vi "Estrazione.vi"(0 "Percorso file invenduti (se vuoto finestra di dialogo)":path) -> (1 "Ci sono numeri estratti invenduti!!!":bool, 2 "Numeri estratti":i32[](array[numeric]))   [LabVIEW 2012]
uses:
  <vilib>/Utility/file.llb/Write To Spreadsheet File (I64).vi
  <vilib>/Utility/file.llb/Read From Spreadsheet File (I64).vi
panel:
  in  "Numero massimo\nvenduto":i32=5000
  in  "Quanti numeri estrarre":i32=25
  out "Numeri invenduti":i64[](array[numeric])
  out "Numeri estratti senza\ncontrollo":i32[](array[numeric]) format="%#.0f"
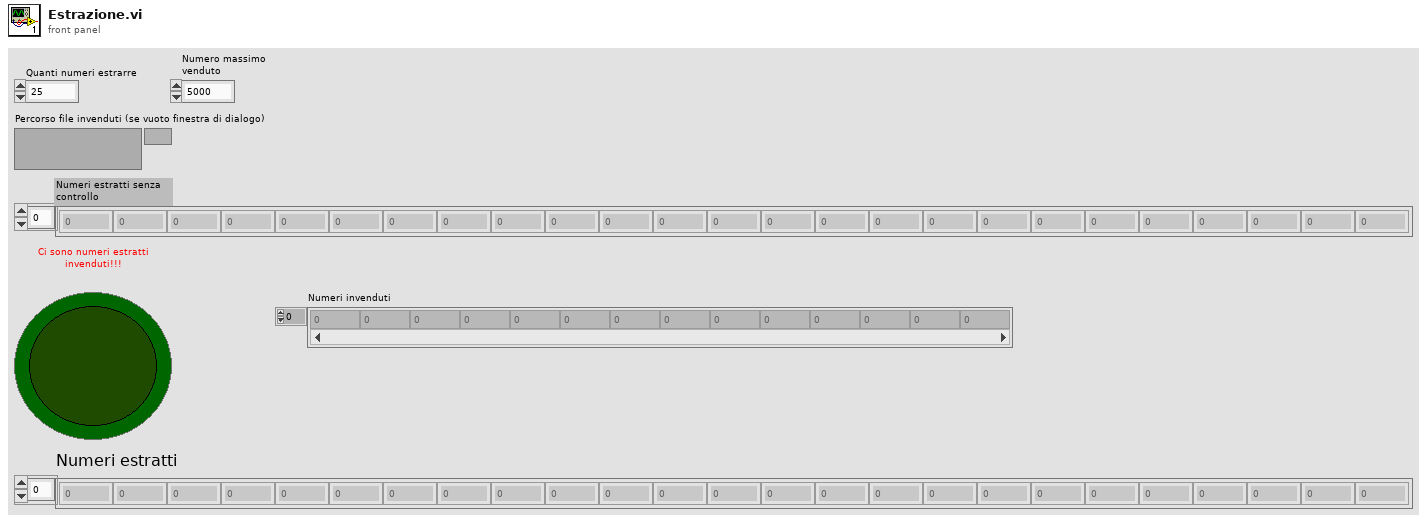
[diagram p1: front panel]
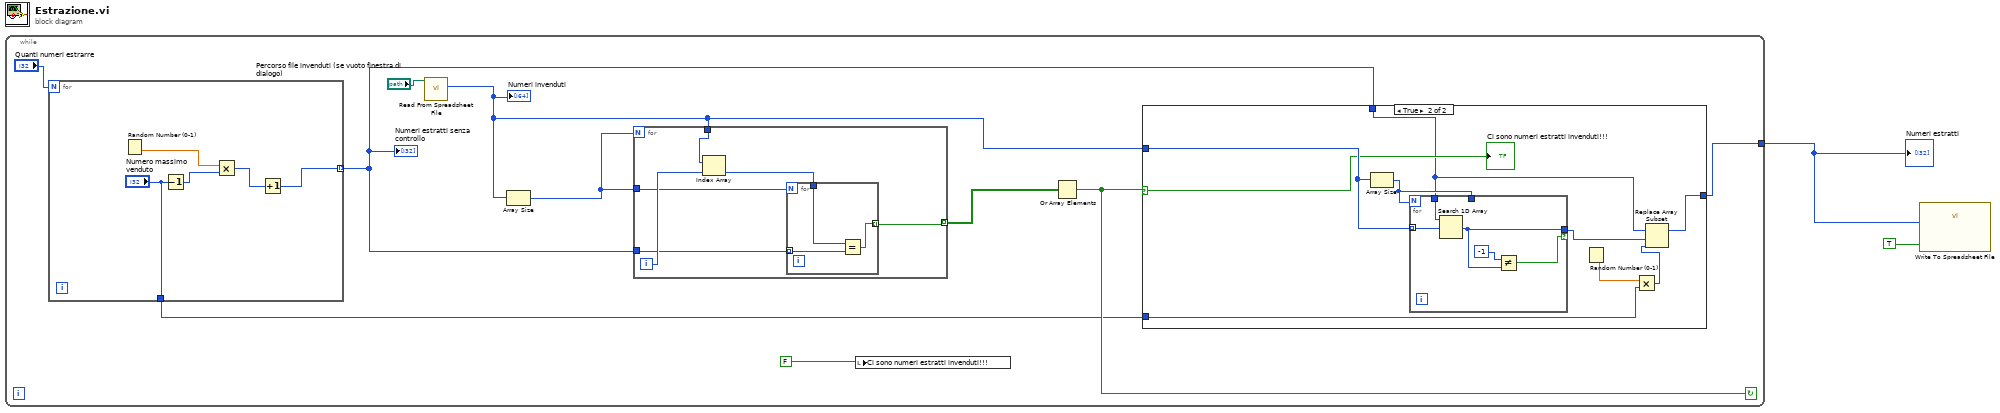
[diagram p0: block diagram]
diagram:
  n1 = while {
    tunnel: [w8] -> w1
    stop <- w7 continue-if-true
    n2 = for {
      N: "Quanti numeri estrarre" -> [_]
      tunnel: [w39] -> w6 mode=indexing
      tunnel: ["Numero massimo\nvenduto"] -> w3
      n3 = Random Number (0-1)() -> (number: 0 to 1=w41:dbl)
      n4 = Decrement(x="Numero massimo\nvenduto") -> (x-1=w38:i32)
      n5 = Multiply(x=w41, y=w38) -> (x*y=w40:i32)
      n6 = Increment(x=w40) -> (x+1=w39:i32)
    }
    "Numeri estratti senza\ncontrollo" <- w6
    n7 = call-poly <vilib>:"Read From Spreadsheet File.vi"("file path (dialog if empty)"="Percorso file invenduti (se vuoto finestra di dialogo)") -> ("first row"=w12:i64[])  [unwired: 6 in, 4 out]
    "Numeri invenduti" <- w12
    n8 = Array Size(array=w12) -> (size(s)=w10:i32)
    n9 = for {
      N: w10 -> [_]
      tunnel: w12 -> [w33]
      tunnel: [w30] -> w9 mode=indexing
      tunnel: w6 -> [w29]
      tunnel: w10 -> [w28]
      i -> [w32]
      n10 = Index Array(array=w33, index=w32) -> (element=w31:i64)
      n11 = for {
        N: w28 -> [_]
        tunnel: w31 -> [w36]
        tunnel: [w35] -> w30 mode=indexing
        tunnel: w29 -> [w34] mode=indexing
        n12 = Equal?(x=w36, y=w34) -> (x = y?=w35:bool)
      }
    }
    n13 = local write "Ci sono numeri estratti invenduti!!!"(FALSE) -> ()
    n14 = Or Array Elements(Boolean array=w9) -> (logical OR=w7:bool)
    n15 = case shown="True" w7 {
      selector: w7 -> [_ w20]
      tunnel: w6 -> [w13 w18]
      tunnel: [w13 w17] -> w8
      tunnel: w12 -> [_ w22]
      tunnel: w3 -> [_ w14]
      frame False {
      }
      frame True {
        n16 = Array Size(array=w22) -> (size(s)=w21:i32)
        n17 = for {
          N: w21 -> [_]
          tunnel: w22 -> [w27] mode=indexing
          tunnel: w18 -> [w26]
          tunnel: w21 -> [_]
          tunnel: [w24] -> w19 if=w23
          n18 = Search 1D Array(1D array=w26, element=w27) -> (index of element=w24:i32)  [unwired: 1 in]
          n19 = Not Equal?(x=-1, y=w24) -> (x != y?=w23:bool)
        }
        n20 = Random Number (0-1)() -> (number: 0 to 1=w16:dbl)
        n21 = Multiply(x=w16, y=w14) -> (x*y=w15:i32)
        n22 = Replace Array Subset(array=w18, new element=w15, index=w19) -> (w17:i32[])
        "Ci sono numeri estratti invenduti!!!" <- w20
      }
    }
  }
  "Numeri estratti" <- w1
  n23 = call-poly <vilib>:"Write To Spreadsheet File.vi"("transpose? (no:F)"=TRUE, "1D data"=w1) -> ()  [unwired: 6 in, 1 out]
